vi "Manufacturer flags DSP402.vi"(4 "Bit 15":T1 items=["---", "OFF", "ON"], 6 "Bit 13":T1 items=["---", "OFF", "ON"], 7 "Bit 14":T1 items=["---", "OFF", "ON"], 8 "error in (no error)":errorcluster, 9 "Bit 12":T1 items=["---", "OFF", "ON"], 10 "Bit 11":T1 items=["---", "OFF", "ON"], 11 "DSP402 in":refnum<class "DSP402.lvclass">) -> (0 "error out":errorcluster, 3 "DSP402 out":refnum<class "DSP402.lvclass">)   [LabVIEW 2024, in "canopen.lvlib" / "DSP402.lvclass"]
uses:
  DSP402.lvclass
  types/threestateFlag.ctl
  canopen.lvlib
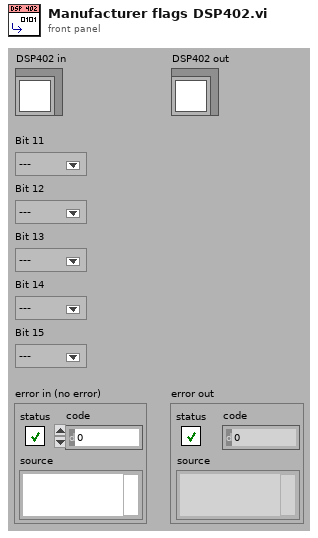
[diagram p1: front panel]
types:
  T1 = typedef "canopen.lvlib/threestateFlag.ctl" = i8
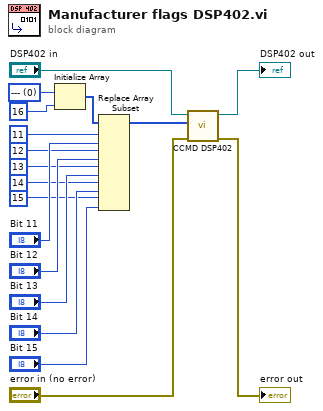
[diagram p0: block diagram]
diagram:
  w13 = T1 0 items=["---", "OFF", "ON"] ("New value")
  n1 = Initialize Array(w13, 16 ("dimension size")) -> (w12:T1[])
  n2 = Replace Array Subset(array=w12, new element #1="Bit 11", index #1=11 ("index"), new element #2="Bit 12", index #2=12 ("index"), new element #3="Bit 13", index #3=13 ("index"), new element #4="Bit 14", index #4=14 ("index"), new element #5="Bit 15", index #5=15 ("index")) -> (w3:T1[])
  n3 = call "CCMD DSP402.vi"("error in (no error)"="error in (no error)", "Mask"=w3, "DSP402 in"="DSP402 in") -> ("error out"=→"error out":errorcluster, "DSP402 out"=→"DSP402 out":refnum<class "DSP402.lvclass">)  [unwired: 3 out]
